vi "PCO_SetHWIOSignal.vi"(8 "error in (no error)":errorcluster {"code" format="%x"}, 9 "strSignal":T1, 10 "wSignalNum":u16, 11 "ph":u64) -> (0 "error out":errorcluster {"code" format="%x"}, 2 "ErrorMessage":i32 format="%x", 3 "ph out":u64)   [LabVIEW 2020, in "SDK.lvlib" / "TimingControl.lvlib"]
doc: "<b>Description:</b>\nThis function does select the settings of a distinct hardware IO signal line. To query the settings of a distinct signal line please use PCO_GetHWIOSignal.\nTo determine the available options for each signal line use PCO_GetHWIOSignalDescriptor.\n\n<b>Supported camera type:</b>\npco.edge, pco.dimax\n\n<b>Descriptor dependency:</b>\ndwGeneralCapsDESC1: HW_IO_SIGNAL_DESCRIPTOR"
uses:
  TimingControl.lvlib
  Structures.lvlib
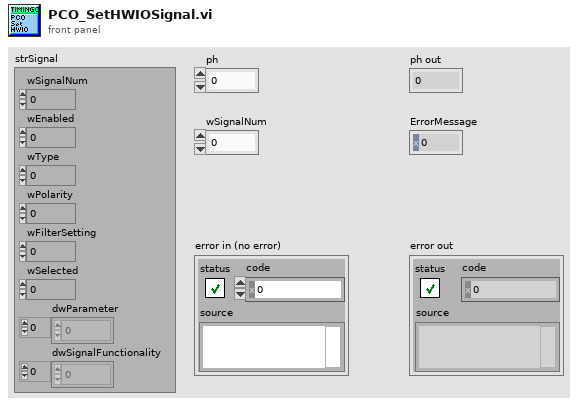
[diagram p1: front panel]
types:
  T1 = cluster{"wSignalNum":u16, "wEnabled":u16, "wType":u16, "wPolarity":u16, "wFilterSetting":u16, "wSelected":u16, "dwParameter":u32[], "dwSignalFunctionality":u32[]}
  T2 = cluster{"wSize":u16, "wSignalNum":u16, "wEnabled":u16, "wType":u16, "wPolarity":u16, "wFilterSetting":u16, "wSelected":u16, "ZZwReserved":u16, "dwParameter":cluster{u32, u32, u32, u32}, "dwSignalFunctionality":cluster{u32, u32, u32, u32}, "ZZdwReserved":cluster{u32, u32, u32}}
  T3 = cluster{"dwParameter[0]":u32, "dwParameter[1]":u32, "dwParameter[2]":u32, "dwParameter[3]":u32}
  T4 = cluster{"dwSignalFunctionality[0]":u32, "dwSignalFunctionality[1]":u32, "dwSignalFunctionality[2]":u32, "dwSignalFunctionality[3]":u32}
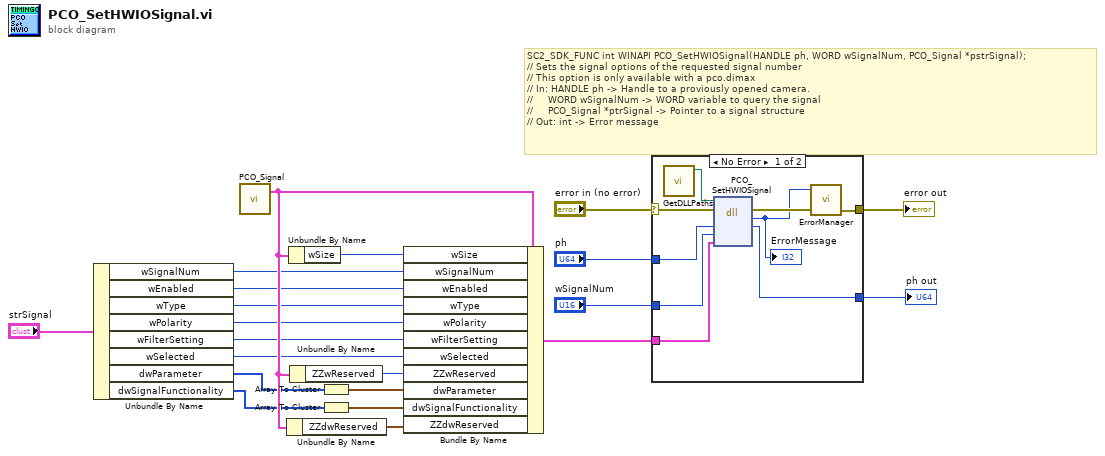
[diagram p0: block diagram]
diagram:
  # "SC2_SDK_FUNC int WINAPI PCO_SetHWIOSignal(HANDLE ph, WORD wSignalNum, PCO_Signal *pstrSignal);\n// Sets the signal options of the requested signal number\n// This option is only available with a pco.dimax\n// In: HANDLE ph -> Handle to a proviously opened camera.\n//     WORD wSignalNum -> WORD variable to query the signal\n//     PCO_Signal *ptrSignal -> Pointer to a signal structure\n// Out: int -> Error message"
  n1 = Unbundle By Name("strSignal") -> ("wSignalNum"=w11:u16, "wEnabled"=w10:u16, "wType"=w9:u16, "wPolarity"=w8:u16, "wFilterSetting"=w7:u16, "wSelected"=w6:u16, "dwParameter"=w5:u32[], "dwSignalFunctionality"=w3:u32[])
  n2 = call "PCO_Signal.vi"() -> ("PCO_Signal_Raw"=w13:T2)  [unwired: 4 in, 3 out]
  n3 = Unbundle By Name(w13) -> ("ZZdwReserved"=w12:cluster{u32, u32, u32})
  n4 = Unbundle By Name(w13) -> ("wSize"=w15:u16)
  n5 = Unbundle By Name(w13) -> ("ZZwReserved"=w14:u16)
  n6 = Array To Cluster(array=w5) -> (cluster=w4:T3)
  n7 = Array To Cluster(array=w3) -> (cluster=w2:T4)
  n8 = Bundle By Name(cluster=w13, "wSize"=w15, "wSignalNum"=w11, "wEnabled"=w10, "wType"=w9, "wPolarity"=w8, "wFilterSetting"=w7, "wSelected"=w6, "ZZwReserved"=w14, "dwParameter"=w4, "dwSignalFunctionality"=w2, "ZZdwReserved"=w12) -> (w1:T2)
  n9 = case shown="No Error" "error in (no error)" {
    selector: "error in (no error)" -> [w26 w32]
    tunnel: "ph" -> [w30 w31]
    tunnel: [w29 w31] -> w20
    tunnel: "wSignalNum" -> [w28 _]
    tunnel: w1 -> [w27 _]
    tunnel: [w24 w32] -> w18
    frame No Error {
      n10 = call "GetDLLPaths.vi"() -> ("SC2_Cam_Path"=w22:path)  [unwired: 9 in, 2 out]
      n11 = dll-call lib="?" fn="PCO_SetHWIOSignal"(path in=w22, error in=w26, "ph"=w30, "wSignalNum"=w28, "pstrSignal"=w27) -> (error out=w25:errorcluster, "return type"=w23:i32, "ph"=w29:u64)  [unwired: 3 in, 1 out]
      "ErrorMessage" <- w23
      n12 = call "ErrorManager.vi"("error in (no error)"=w25, "error code"=w23) -> ("error out"=w24:errorcluster)  [unwired: 3 in]
    }
    frame Error {
    }
  }
  "ph out" <- w20
  "error out" <- w18
